vi "tsfifo_disable_receive_fifo.vi"(8 "error in (no error)":errorcluster, 11 "Path":path) -> (0 "error out":errorcluster, 3 "Path output":path)   [LabVIEW 2014]
doc: "The function name is void tsFifoduisable_deceive_fifo();\nFunction introduction: Disable the internal receiving cache mechanism of the driver\nWhen the user does not need to receive the message by reading the cache, call this function to close it\nInternal cache.\nNo input parameters\nNo return value"
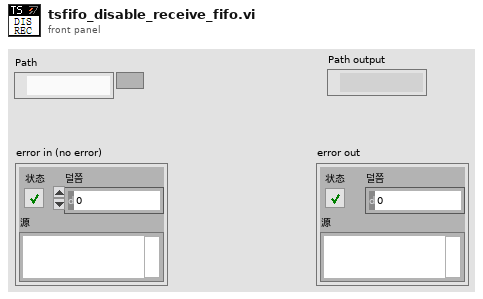
[diagram p1: front panel]
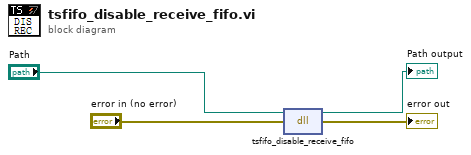
[diagram p0: block diagram]
diagram:
  n1 = dll-call lib="D:/Program Files (x86)/TOSUN/TSMaster/Data/SDK/lib/x86/TSMaster.dll" fn="tsfifo_disable_receive_fifo"(path in="Path", error in="error in (no error)") -> (path out=→"Path output":path, error out=→"error out":errorcluster)  [unwired: 2 in]
